vi "E_Stop_Local_Read_INI_Sub_VI.vi"(8 "error in (no error)":errorcluster, 11 "Config File Path":path=path "\\\\Ultrasonic_Test_Scripts\\Build/UltraSonic_Test_Scripts/BF_INT_FirmWareUpgrade_Auto/FirmwareUpgrade_Test/FirmwareUpgrade_Test_Config.ini") -> (2 "E-stop Parameters":T1)   [LabVIEW 2017]
uses:
  <vilib>/Utility/config.llb/Read Key (I32).vi
  <vilib>/Utility/config.llb/Read Key (String).vi
  <vilib>/Utility/config.llb/Read Key (Path).vi
  <vilib>/Utility/config.llb/NI_LVConfig.lvlib
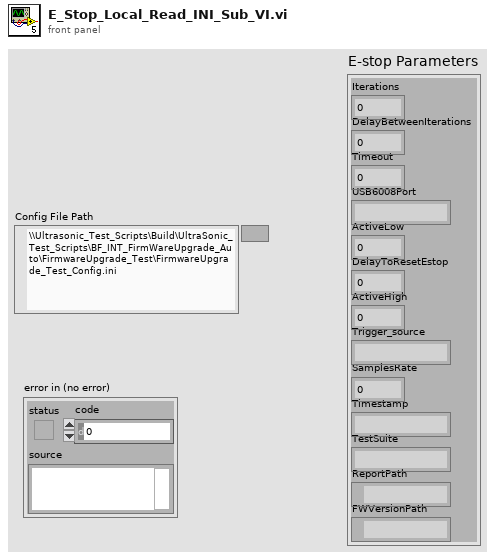
[diagram p1: front panel]
types:
  T1 = cluster{"Iterations":u32, "DelayBetweenIterations":u32, "Timeout":u32, "USB6008Port":string, "ActiveLow":i32, "DelayToResetEstop":i32, "ActiveHigh":i32, "Trigger_source":string, "SamplesRate":i32, "Timestamp":string, "TestSuite":string, "ReportPath":path, "FWVersionPath":path}
  T2 = typedef "NI_LVConfig.lvlib/Config Data RefNum.ctl" = refnum<k1>
  T3 = cluster{u32, u32, u32, "value":string, i32, i32, "value":i32, "value":string, i32, "value":string, "value":string, "value":path, path}
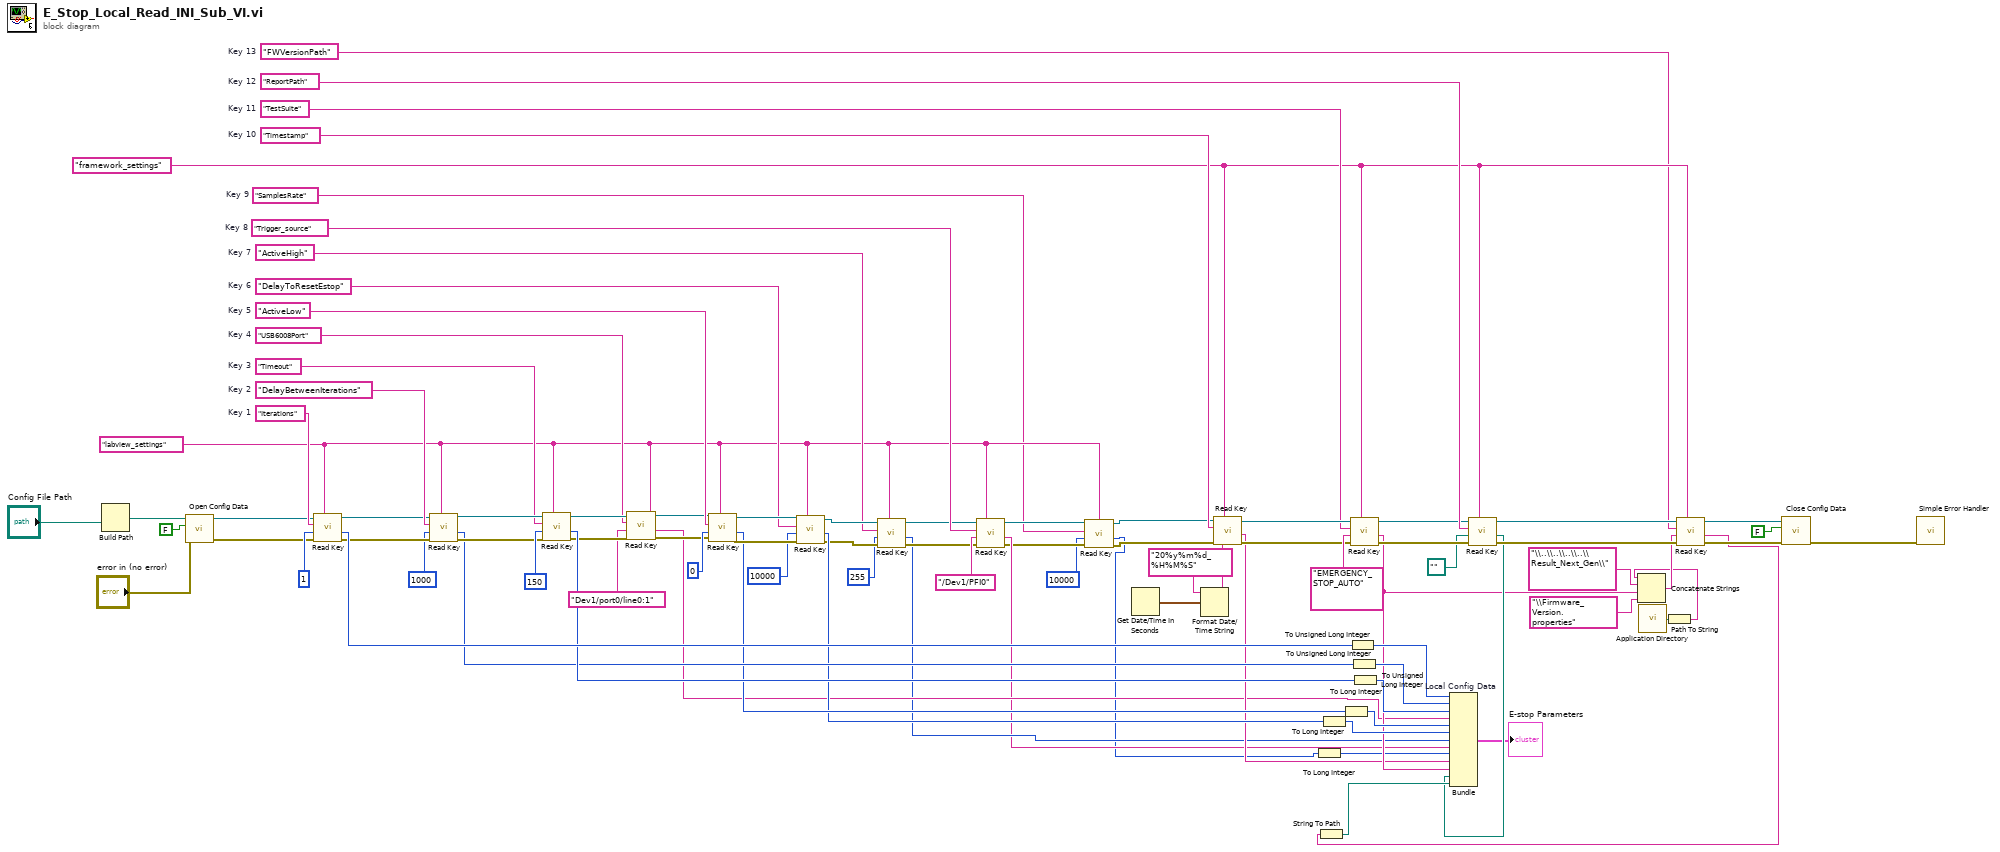
[diagram p0: block diagram]
diagram:
  w7 = "SamplesRate"  # Key 9
  w27 = "Trigger_source"  # Key 8
  w14 = "ActiveHigh"  # Key 7
  w39 = "DelayToResetEstop"  # Key 6
  w40 = "ActiveLow"  # Key 5
  w21 = "USB6008Port"  # Key 4
  w54 = "FWVersionPath"  # Key 13
  w66 = "Timestamp"  # Key 10
  w61 = "TestSuite"  # Key 11
  w67 = "Timeout"  # Key 3
  w76 = "ReportPath"  # Key 12
  w81 = "DelayBetweenIterations"  # Key 2
  w83 = "Iterations"  # Key 1
  w55 = "framework_settings" ("section")
  w8 = "labview_settings" ("section")
  n1 = Build Path(name or relative path="Config File Path") -> (appended path=w85:path)  [unwired: 1 in]
  n2 = call <vilib>:"Open Config Data.vi"("error in (no error)"="error in (no error)", "create file if necessary (T)"=FALSE ("create file if necessary? (T)"), "configuration file path"=w85) -> ("error out"=w48:errorcluster, "refnum"=w47:T2)  [unwired: 6 in, 1 out]
  n3 = call-poly <vilib>:"Read Key.vi"("section"=w8, "error in (no error)"=w48, "default value"=1, "key"=w83, "refnum"=w47) -> ("error out"=w79:errorcluster, "value"=w82:i32, "refnum out"=w80:T2)  [unwired: 4 out]
  n4 = call-poly <vilib>:"Read Key.vi"("section"=w8, "error in (no error)"=w79, "default value"=1000, "key"=w81, "refnum"=w80) -> ("error out"=w74:errorcluster, "value"=w46:i32, "refnum out"=w73:T2)  [unwired: 4 out]
  n5 = call-poly <vilib>:"Read Key.vi"("section"=w8, "error in (no error)"=w74, "default value"=150, "key"=w67, "refnum"=w73) -> ("error out"=w23:errorcluster, "value"=w71:i32, "refnum out"=w25:T2)  [unwired: 4 out]
  n6 = call-poly <vilib>:"Read Key.vi"("section"=w8, "error in (no error)"=w23, "default value"="Dev1/port0/line0:1", "key"=w21, "refnum"=w25) -> ("error out"=w22:errorcluster, "value"=w19:string, "refnum out"=w24:T2)  [unwired: 1 in, 3 out]
  n7 = call-poly <vilib>:"Read Key.vi"("section"=w8, "error in (no error)"=w22, "default value"=0, "key"=w40, "refnum"=w24) -> ("error out"=w44:errorcluster, "value"=w42:i32, "refnum out"=w45:T2)  [unwired: 4 out]
  n8 = call-poly <vilib>:"Read Key.vi"("section"=w8, "error in (no error)"=w44, "default value"=10000, "key"=w39, "refnum"=w45) -> ("error out"=w16:errorcluster, "value"=w41:i32, "refnum out"=w18:T2)  [unwired: 4 out]
  n9 = call-poly <vilib>:"Read Key.vi"("section"=w8, "error in (no error)"=w16, "default value"=255, "key"=w14, "refnum"=w18) -> ("error out"=w15:errorcluster, "value"=w12:i32, "refnum out"=w17:T2)  [unwired: 4 out]
  n10 = call-poly <vilib>:"Read Key.vi"("section"=w8, "error in (no error)"=w15, "default value"="/Dev1/PFI0", "key"=w27, "refnum"=w17) -> ("error out"=w9:errorcluster, "value"=w11:string, "refnum out"=w10:T2)  [unwired: 1 in, 3 out]
  n11 = call-poly <vilib>:"Read Key.vi"("section"=w8, "error in (no error)"=w9, "default value"=10000, "key"=w7, "refnum"=w10) -> ("error out"=w4:errorcluster, "value"=w3:i32, "refnum out"=w5:T2)  [unwired: 4 out]
  n12 = Get Date/Time In Seconds() -> (seconds since 1Jan1904=w68:timestamp)
  n13 = Format Date/Time String(time format string (%c)="20%y%m%d_%H%M%S", seconds (now)=w68) -> (date/time string=w69:string)  [unwired: 1 out]
  n14 = call-poly <vilib>:"Read Key.vi"("section"=w55, "error in (no error)"=w4, "default value"=w69, "key"=w66, "refnum"=w5) -> ("error out"=w63:errorcluster, "value"=w29:string, "refnum out"=w64:T2)  [unwired: 1 in, 3 out]
  n15 = To Long Integer(number=w3) -> (32bit integer=w2:i32)
  n16 = To Long Integer(number=w41) -> (32bit integer=w36:i32)
  n17 = To Long Integer(number=w42) -> (32bit integer=w43:i32)
  n18 = To Unsigned Long Integer(number=w82) -> (unsigned 32bit integer=w89:u32)
  n19 = call-poly <vilib>:"Read Key.vi"("section"=w55, "error in (no error)"=w63, "default value"="EMERGENCY_STOP_AUTO", "key"=w61, "refnum"=w64) -> ("error out"=w62:errorcluster, "value"=w30:string, "refnum out"=w65:T2)  [unwired: 1 in, 3 out]
  n20 = To Unsigned Long Integer(number=w46) -> (unsigned 32bit integer=w35:u32)
  n21 = To Unsigned Long Integer(number=w71) -> (unsigned 32bit integer=w34:u32)
  n22 = call-poly <vilib>:"Read Key.vi"("section"=w55, "error in (no error)"=w62, "default value"=path "", "key"=w76, "refnum"=w65) -> ("error out"=w56:errorcluster, "value"=w31:path, "refnum out"=w59:T2)  [unwired: 1 in, 3 out]
  n23 = call <vilib>:"Application Directory.vi"() -> ("Application Directory"=w50:path)
  n24 = Path To String(path=w50) -> (string=w49:string)
  n25 = Concatenate Strings(w49, "\\..\\..\\..\\..\\Result_Next_Gen\\" ("default value"), w30, "\\Firmware_Version.properties" ("default value")) -> (w53:string)
  n26 = call-poly <vilib>:"Read Key.vi"("section"=w55, "error in (no error)"=w56, "default value"=w53, "key"=w54, "refnum"=w59) -> ("error out"=w57:errorcluster, "value"=w33:string, "refnum out"=w58:T2)  [unwired: 1 in, 3 out]
  n27 = String To Path(string=w33) -> (path=w32:path)
  n28 = Bundle "Local Config Data"(w89, w35, w34, "value"=w19, w43, w36, "value"=w12, "value"=w11, w2, "value"=w29, "value"=w30, "value"=w31, w32) -> (→"E-stop Parameters":T3)  [unwired: 1 in]
  n29 = call <vilib>:"Close Config Data.vi"("error in (no error)"=w57, "write file if changed (T)"=FALSE ("write configuration file? (T)"), "refnum"=w58) -> ("error out"=w86:errorcluster)  [unwired: 8 out]
  n30 = call <vilib>:"Simple Error Handler.vi"("error in (no error)"=w86) -> ()  [unwired: 1 in, 8 out]
